vi "FipsAdjacent.vi"() -> (11 "Fips":i32[](array[numeric]))   [LabVIEW 2017] (continued)
40035\t\"Labette County, KS\"\t20099\n\"Craig County, OK\"\t40035\t\"Craig County, OK\"\t40035\n\"Craig County, OK\"\t40035\t\"Delaware County, OK\"\t40041\n\"Craig County, OK\"\t40035\t\"Mayes County, OK\"\t40097\n\"Craig County, OK\"\t40035\t\"Nowata County, OK\"\t40105\n\"Craig County, OK\"\t40035\t\"Ottawa County, OK\"\t40115\n\"Craig County, OK\"\t40035\t\"Rogers County, OK\"\t40131\n\"Creek County, OK\"\t40037\t\"Creek County, OK\"\t40037\n\"Creek County, OK\"\t40037\t\"Lincoln County, OK\"\t40081\n\"Creek County, OK\"\t40037\t\"Okfuskee County, OK\"\t40107\n\"Creek County, OK\"\t40037\t\"Okmulgee County, OK\"\t40111\n\"Creek County, OK\"\t40037\t\"Pawnee County, OK\"\t40117\n\"Creek County, OK\"\t40037\t\"Payne County, OK\"\t40119\n\"Creek County, OK\"\t40037\t\"Tulsa County, OK\"\t40143\n\"Custer County, OK\"\t40039\t\"Beckham County, OK\"\t40009\n\"Custer County, OK\"\t40039\t\"Blaine County, OK\"\t40011\n\"Custer County, OK\"\t40039\t\"Caddo County, OK\"\t40015\n\"Custer County, OK\"\t40039\t\"Custer County, OK\"\t40039\n\"Custer County, OK\"\t40039\t\"Dewey County, OK\"\t40043\n\"Custer County, OK\"\t40039\t\"Roger Mills County, OK\"\t40129\n\"Custer County, OK\"\t40039\t\"Washita County, OK\"\t40149\n\"Delaware County, OK\"\t40041\t\"Benton County, AR\"\t05007\n\"Delaware County, OK\"\t40041\t\"McDonald County, MO\"\t29119\n\"Delaware County, OK\"\t40041\t\"Adair County, OK\"\t40001\n\"Delaware County, OK\"\t40041\t\"Cherokee County, OK\"\t40021\n\"Delaware County, OK\"\t40041\t\"Craig County, OK\"\t40035\n\"Delaware County, OK\"\t40041\t\"Delaware County, OK\"\t40041\n\"Delaware County, OK\"\t40041\t\"Mayes County, OK\"\t40097\n\"Delaware County, OK\"\t40041\t\"Ottawa County, OK\"\t40115\n\"Dewey County, OK\"\t40043\t\"Blaine County, OK\"\t40011\n\"Dewey County, OK\"\t40043\t\"Custer County, OK\"\t40039\n\"Dewey County, OK\"\t40043\t\"Dewey County, OK\"\t40043\n\"Dewey County, OK\"\t40043\t\"Ellis County, OK\"\t40045\n\"Dewey County, OK\"\t40043\t\"Major County, OK\"\t40093\n\"Dewey County, OK\"\t40043\t\"Roger Mills County, OK\"\t40129\n\"Dewey County, OK\"\t40043\t\"Woodward County, OK\"\t40153\n\"Ellis County, OK\"\t40045\t\"Beaver County, OK\"\t40007\n\"Ellis County, OK\"\t40045\t\"Dewey County, OK\"\t40043\n\"Ellis County, OK\"\t40045\t\"Ellis County, OK\"\t40045\n\"Ellis County, OK\"\t40045\t\"Harper County, OK\"\t40059\n\"Ellis County, OK\"\t40045\t\"Roger Mills County, OK\"\t40129\n\"Ellis County, OK\"\t40045\t\"Woodward County, OK\"\t40153\n\"Ellis County, OK\"\t40045\t\"Hemphill County, TX\"\t48211\n\"Ellis County, OK\"\t40045\t\"Lipscomb County, TX\"\t48295\n\"Garfield County, OK\"\t40047\t\"Alfalfa County, OK\"\t40003\n\"Garfield County, OK\"\t40047\t\"Garfield County, OK\"\t40047\n\"Garfield County, OK\"\t40047\t\"Grant County, OK\"\t40053\n\"Garfield County, OK\"\t40047\t\"Kay County, OK\"\t40071\n\"Garfield County, OK\"\t40047\t\"Kingfisher County, OK\"\t40073\n\"Garfield County, OK\"\t40047\t\"Logan County, OK\"\t40083\n\"Garfield County, OK\"\t40047\t\"Major County, OK\"\t40093\n\"Garfield County, OK\"\t40047\t\"Noble County, OK\"\t40103\n\"Garvin County, OK\"\t40049\t\"Carter County, OK\"\t40019\n\"Garvin County, OK\"\t40049\t\"Garvin County, OK\"\t40049\n\"Garvin County, OK\"\t40049\t\"Grady County, OK\"\t40051\n\"Garvin County, OK\"\t40049\t\"McClain County, OK\"\t40087\n\"Garvin County, OK\"\t40049\t\"Murray County, OK\"\t40099\n\"Garvin County, OK\"\t40049\t\"Pontotoc County, OK\"\t40123\n\"Garvin County, OK\"\t40049\t\"Stephens County, OK\"\t40137\n\"Grady County, OK\"\t40051\t\"Caddo County, OK\"\t40015\n\"Grady County, OK\"\t40051\t\"Canadian County, OK\"\t40017\n\"Grady County, OK\"\t40051\t\"Comanche County, OK\"\t40031\n\"Grady County, OK\"\t40051\t\"Garvin County, OK\"\t40049\n\"Grady County, OK\"\t40051\t\"Grady County, OK\"\t40051\n\"Grady County, OK\"\t40051\t\"McClain County, OK\"\t40087\n\"Grady County, OK\"\t40051\t\"Stephens County, OK\"\t40137\n\"Grant County, OK\"\t40053\t\"Harper County, KS\"\t20077\n\"Grant County, OK\"\t40053\t\"Sumner County, KS\"\t20191\n\"Grant County, OK\"\t40053\t\"Alfalfa County, OK\"\t40003\n\"Grant County, OK\"\t40053\t\"Garfield County, OK\"\t40047\n\"Grant County, OK\"\t40053\t\"Grant County, OK\"\t40053\n\"Grant County, OK\"\t40053\t\"Kay County, OK\"\t40071\n\"Greer County, OK\"\t40055\t\"Beckham County, OK\"\t40009\n\"Greer County, OK\"\t40055\t\"Greer County, OK\"\t40055\n\"Greer County, OK\"\t40055\t\"Harmon County, OK\"\t40057\n\"Greer County, OK\"\t40055\t\"Jackson County, OK\"\t40065\n\"Greer County, OK\"\t40055\t\"Kiowa County, OK\"\t40075\n\"Harmon County, OK\"\t40057\t\"Beckham County, OK\"\t40009\n\"Harmon County, OK\"\t40057\t\"Greer County, OK\"\t40055\n\"Harmon County, OK\"\t40057\t\"Harmon County, OK\"\t40057\n\"Harmon County, OK\"\t40057\t\"Jackson County, OK\"\t40065\n\"Harmon County, OK\"\t40057\t\"Childress County, TX\"\t48075\n\"Harmon County, OK\"\t40057\t\"Collingsworth County, TX\"\t48087\n\"Harmon County, OK\"\t40057\t\"Hardeman County, TX\"\t48197\n\"Harper County, OK\"\t40059\t\"Clark County, KS\"\t20025\n\"Harper County, OK\"\t40059\t\"Comanche County, KS\"\t20033\n\"Harper County, OK\"\t40059\t\"Beaver County, OK\"\t40007\n\"Harper County, OK\"\t40059\t\"Ellis County, OK\"\t40045\n\"Harper County, OK\"\t40059\t\"Harper County, OK\"\t40059\n\"Harper County, OK\"\t40059\t\"Woods County, OK\"\t40151\n\"Harper County, OK\"\t40059\t\"Woodward County, OK\"\t40153\n\"Haskell County, OK\"\t40061\t\"Haskell County, OK\"\t40061\n\"Haskell County, OK\"\t40061\t\"Latimer County, OK\"\t40077\n\"Haskell County, OK\"\t40061\t\"Le Flore County, OK\"\t40079\n\"Haskell County, OK\"\t40061\t\"McIntosh County, OK\"\t40091\n\"Haskell County, OK\"\t40061\t\"Muskogee County, OK\"\t40101\n\"Haskell County, OK\"\t40061\t\"Pittsburg County, OK\"\t40121\n\"Haskell County, OK\"\t40061\t\"Sequoyah County, OK\"\t40135\n\"Hughes County, OK\"\t40063\t\"Coal County, OK\"\t40029\n\"Hughes County, OK\"\t40063\t\"Hughes County, OK\"\t40063\n\"Hughes County, OK\"\t40063\t\"McIntosh County, OK\"\t40091\n\"Hughes County, OK\"\t40063\t\"Okfuskee County, OK\"\t40107\n\"Hughes County, OK\"\t40063\t\"Pittsburg County, OK\"\t40121\n\"Hughes County, OK\"\t40063\t\"Pontotoc County, OK\"\t40123\n\"Hughes County, OK\"\t40063\t\"Seminole County, OK\"\t40133\n\"Jackson County, OK\"\t40065\t\"Greer County, OK\"\t40055\n\"Jackson County, OK\"\t40065\t\"Harmon County, OK\"\t40057\n\"Jackson County, OK\"\t40065\t\"Jackson County, OK\"\t40065\n\"Jackson County, OK\"\t40065\t\"Kiowa County, OK\"\t40075\n\"Jackson County, OK\"\t40065\t\"Tillman County, OK\"\t40141\n\"Jackson County, OK\"\t40065\t\"Hardeman County, TX\"\t48197\n\"Jackson County, OK\"\t40065\t\"Wilbarger County, TX\"\t48487\n\"Jefferson County, OK\"\t40067\t\"Carter County, OK\"\t40019\n\"Jefferson County, OK\"\t40067\t\"Cotton County, OK\"\t40033\n\"Jefferson County, OK\"\t40067\t\"Jefferson County, OK\"\t40067\n\"Jefferson County, OK\"\t40067\t\"Love County, OK\"\t40085\n\"Jefferson County, OK\"\t40067\t\"Stephens County, OK\"\t40137\n\"Jefferson County, OK\"\t40067\t\"Clay County, TX\"\t48077\n\"Jefferson County, OK\"\t40067\t\"Montague County, TX\"\t48337\n\"Johnston County, OK\"\t40069\t\"Atoka County, OK\"\t40005\n\"Johnston County, OK\"\t40069\t\"Bryan County, OK\"\t40013\n\"Johnston County, OK\"\t40069\t\"Carter County, OK\"\t40019\n\"Johnston County, OK\"\t40069\t\"Coal County, OK\"\t40029\n\"Johnston County, OK\"\t40069\t\"Johnston County, OK\"\t40069\n\"Johnston County, OK\"\t40069\t\"Marshall County, OK\"\t40095\n\"Johnston County, OK\"\t40069\t\"Murray County, OK\"\t40099\n\"Johnston County, OK\"\t40069\t\"Pontotoc County, OK\"\t40123\n\"Kay County, OK\"\t40071\t\"Cowley County, KS\"\t20035\n\"Kay County, OK\"\t40071\t\"Sumner County, KS\"\t20191\n\"Kay County, OK\"\t40071\t\"Garfield County, OK\"\t40047\n\"Kay County, OK\"\t40071\t\"Grant County, OK\"\t40053\n\"Kay County, OK\"\t40071\t\"Kay County, OK\"\t40071\n\"Kay County, OK\"\t40071\t\"Noble County, OK\"\t40103\n\"Kay County, OK\"\t40071\t\"Osage County, OK\"\t40113\n\"Kingfisher County, OK\"\t40073\t\"Blaine County, OK\"\t40011\n\"Kingfisher County, OK\"\t40073\t\"Canadian County, OK\"\t40017\n\"Kingfisher County, OK\"\t40073\t\"Garfield County, OK\"\t40047\n\"Kingfisher County, OK\"\t40073\t\"Kingfisher County, OK\"\t40073\n\"Kingfisher County, OK\"\t40073\t\"Logan County, OK\"\t40083\n\"Kingfisher County, OK\"\t40073\t\"Major County, OK\"\t40093\n\"Kingfisher County, OK\"\t40073\t\"Oklahoma County, OK\"\t40109\n\"Kiowa County, OK\"\t40075\t\"Beckham County, OK\"\t40009\n\"Kiowa County, OK\"\t40075\t\"Caddo County, OK\"\t40015\n\"Kiowa County, OK\"\t40075\t\"Comanche County, OK\"\t40031\n\"Kiowa County, OK\"\t40075\t\"Greer County, OK\"\t40055\n\"Kiowa County, OK\"\t40075\t\"Jackson County, OK\"\t40065\n\"Kiowa County, OK\"\t40075\t\"Kiowa County, OK\"\t40075\n\"Kiowa County, OK\"\t40075\t\"Tillman County, OK\"\t40141\n\"Kiowa County, OK\"\t40075\t\"Washita County, OK\"\t40149\n\"Latimer County, OK\"\t40077\t\"Haskell County, OK\"\t40061\n\"Latimer County, OK\"\t40077\t\"Latimer County, OK\"\t40077\n\"Latimer County, OK\"\t40077\t\"Le Flore County, OK\"\t40079\n\"Latimer County, OK\"\t40077\t\"Pittsburg County, OK\"\t40121\n\"Latimer County, OK\"\t40077\t\"Pushmataha County, OK\"\t40127\n\"Le Flore County, OK\"\t40079\t\"Polk County, AR\"\t05113\n\"Le Flore County, OK\"\t40079\t\"Scott County, AR\"\t05127\n\"Le Flore County, OK\"\t40079\t\"Sebastian County, AR\"\t05131\n\"Le Flore County, OK\"\t40079\t\"Haskell County, OK\"\t40061\n\"Le Flore County, OK\"\t40079\t\"Latimer County, OK\"\t40077\n\"Le Flore County, OK\"\t40079\t\"Le Flore County, OK\"\t40079\n\"Le Flore County, OK\"\t40079\t\"McCurtain County, OK\"\t40089\n\"Le Flore County, OK\"\t40079\t\"Pushmataha County, OK\"\t40127\n\"Le Flore County, OK\"\t40079\t\"Sequoyah County, OK\"\t40135\n\"Lincoln County, OK\"\t40081\t\"Creek County, OK\"\t40037\n\"Lincoln County, OK\"\t40081\t\"Lincoln County, OK\"\t40081\n\"Lincoln County, OK\"\t40081\t\"Logan County, OK\"\t40083\n\"Lincoln County, OK\"\t40081\t\"Okfuskee County, OK\"\t40107\n\"Lincoln County, OK\"\t40081\t\"Oklahoma County, OK\"\t40109\n\"Lincoln County, OK\"\t40081\t\"Payne County, OK\"\t40119\n\"Lincoln County, OK\"\t40081\t\"Pottawatomie County, OK\"\t40125\n\"Logan County, OK\"\t40083\t\"Canadian County, OK\"\t40017\n\"Logan County, OK\"\t40083\t\"Garfield County, OK\"\t40047\n\"Logan County, OK\"\t40083\t\"Kingfisher County, OK\"\t40073\n\"Logan County, OK\"\t40083\t\"Lincoln County, OK\"\t40081\n\"Logan County, OK\"\t40083\t\"Logan County, OK\"\t40083\n\"Logan County, OK\"\t40083\t\"Noble County, OK\"\t40103\n\"Logan County, OK\"\t40083\t\"Oklahoma County, OK\"\t40109\n\"Logan County, OK\"\t40083\t\"Payne County, OK\"\t40119\n\"Love County, OK\"\t40085\t\"Carter County, OK\"\t40019\n\"Love County, OK\"\t40085\t\"Jefferson County, OK\"\t40067\n\"Love County, OK\"\t40085\t\"Love County, OK\"\t40085\n\"Love County, OK\"\t40085\t\"Marshall County, OK\"\t40095\n\"Love County, OK\"\t40085\t\"Cooke County, TX\"\t48097\n\"Love County, OK\"\t40085\t\"Grayson County, TX\"\t48181\n\"Love County, OK\"\t40085\t\"Montague County, TX\"\t48337\n\"McClain County, OK\"\t40087\t\"Canadian County, OK\"\t40017\n\"McClain County, OK\"\t40087\t\"Cleveland County, OK\"\t40027\n\"McClain County, OK\"\t40087\t\"Garvin County, OK\"\t40049\n\"McClain County, OK\"\t40087\t\"Grady County, OK\"\t40051\n\"McClain County, OK\"\t40087\t\"McClain County, OK\"\t40087\n\"McClain County, OK\"\t40087\t\"Pontotoc County, OK\"\t40123\n\"McClain County, OK\"\t40087\t\"Pottawatomie County, OK\"\t40125\n\"McCurtain County, OK\"\t40089\t\"Little River County, AR\"\t05081\n\"McCurtain County, OK\"\t40089\t\"Polk County, AR\"\t05113\n\"McCurtain County, OK\"\t40089\t\"Sevier County, AR\"\t05133\n\"McCurtain County, OK\"\t40089\t\"Choctaw County, OK\"\t40023\n\"McCurtain County, OK\"\t40089\t\"Le Flore County, OK\"\t40079\n\"McCurtain County, OK\"\t40089\t\"McCurtain County, OK\"\t40089\n\"McCurtain County, OK\"\t40089\t\"Pushmataha County, OK\"\t40127\n\"McCurtain County, OK\"\t40089\t\"Bowie County, TX\"\t48037\n\"McCurtain County, OK\"\t40089\t\"Red River County, TX\"\t48387\n\"McIntosh County, OK\"\t40091\t\"Haskell County, OK\"\t40061\n\"McIntosh County, OK\"\t40091\t\"Hughes County, OK\"\t40063\n\"McIntosh County, OK\"\t40091\t\"McIntosh County, OK\"\t40091\n\"McIntosh County, OK\"\t40091\t\"Muskogee County, OK\"\t40101\n\"McIntosh County, OK\"\t40091\t\"Okfuskee County, OK\"\t40107\n\"McIntosh County, OK\"\t40091\t\"Okmulgee County, OK\"\t40111\n\"McIntosh County, OK\"\t40091\t\"Pittsburg County, OK\"\t40121\n\"Major County, OK\"\t40093\t\"Alfalfa County, OK\"\t40003\n\"Major County, OK\"\t40093\t\"Blaine County, OK\"\t40011\n\"Major County, OK\"\t40093\t\"Dewey County, OK\"\t40043\n\"Major County, OK\"\t40093\t\"Garfield County, OK\"\t40047\n\"Major County, OK\"\t40093\t\"Kingfisher County, OK\"\t40073\n\"Major County, OK\"\t40093\t\"Major County, OK\"\t40093\n\"Major County, OK\"\t40093\t\"Woods County, OK\"\t40151\n\"Major County, OK\"\t40093\t\"Woodward County, OK\"\t40153\n\"Marshall County, OK\"\t40095\t\"Bryan County, OK\"\t40013\n\"Marshall County, OK\"\t40095\t\"Carter County, OK\"\t40019\n\"Marshall County, OK\"\t40095\t\"Johnston County, OK\"\t40069\n\"Marshall County, OK\"\t40095\t\"Love County, OK\"\t40085\n\"Marshall County, OK\"\t40095\t\"Marshall County, OK\"\t40095\n\"Marshall County, OK\"\t40095\t\"Grayson County, TX\"\t48181\n\"Mayes County, OK\"\t40097\t\"Cherokee County, OK\"\t40021\n\"Mayes County, OK\"\t40097\t\"Craig County, OK\"\t40035\n\"Mayes County, OK\"\t40097\t\"Delaware County, OK\"\t40041\n\"Mayes County, OK\"\t40097\t\"Mayes County, OK\"\t40097\n\"Mayes County, OK\"\t40097\t\"Rogers County, OK\"\t40131\n\"Mayes County, OK\"\t40097\t\"Wagoner County, OK\"\t40145\n\"Murray County, OK\"\t40099\t\"Carter County, OK\"\t40019\n\"Murray County, OK\"\t40099\t\"Garvin County, OK\"\t40049\n\"Murray County, OK\"\t40099\t\"Johnston County, OK\"\t40069\n\"Murray County, OK\"\t40099\t\"Murray County, OK\"\t40099\n\"Murray County, OK\"\t40099\t\"Pontotoc County, OK\"\t40123\n\"Muskogee County, OK\"\t40101\t\"Cherokee County, OK\"\t40021\n\"Muskogee County, OK\"\t40101\t\"Haskell County, OK\"\t40061\n\"Muskogee County, OK\"\t40101\t\"McIntosh County, OK\"\t40091\n\"Muskogee County, OK\"\t40101\t\"Muskogee County, OK\"\t40101\n\"Muskogee County, OK\"\t40101\t\"Okmulgee County, OK\"\t40111\n\"Muskogee County, OK\"\t40101\t\"Sequoyah County, OK\"\t40135\n\"Muskogee County, OK\"\t40101\t\"Wagoner County, OK\"\t40145\n\"Noble County, OK\"\t40103\t\"Garfield County, OK\"\t40047\n\"Noble County, OK\"\t40103\t\"Kay County, OK\"\t40071\n\"Noble County, OK\"\t40103\t\"Logan County, OK\"\t40083\n\"Noble County, OK\"\t40103\t\"Noble County, OK\"\t40103\n\"Noble County, OK\"\t40103\t\"Osage County, OK\"\t40113\n\"Noble County, OK\"\t40103\t\"Pawnee County, OK\"\t40117\n\"Noble County, OK\"\t40103\t\"Payne County, OK\"\t40119\n\"Nowata County, OK\"\t40105\t\"Labette County, KS\"\t20099\n\"Nowata County, OK\"\t40105\t\"Montgomery County, KS\"\t20125\n\"Nowata County, OK\"\t40105\t\"Craig County, OK\"\t40035\n\"Nowata County, OK\"\t40105\t\"Nowata County, OK\"\t40105\n\"Nowata County, OK\"\t40105\t\"Rogers County, OK\"\t40131\n\"Nowata County, OK\"\t40105\t\"Washington County, OK\"\t40147\n\"Okfuskee County, OK\"\t40107\t\"Creek County, OK\"\t40037\n\"Okfuskee County, OK\"\t40107\t\"Hughes County, OK\"\t40063\n\"Okfuskee County, OK\"\t40107\t\"Lincoln County, OK\"\t40081\n\"Okfuskee County, OK\"\t40107\t\"McIntosh County, OK\"\t40091\n\"Okfuskee County, OK\"\t40107\t\"Okfuskee County, OK\"\t40107\n\"Okfuskee County, OK\"\t40107\t\"Okmulgee County, OK\"\t40111\n\"Okfuskee County, OK\"\t40107\t\"Pottawatomie County, OK\"\t40125\n\"Okfuskee County, OK\"\t40107\t\"Seminole County, OK\"\t40133\n\"Oklahoma County, OK\"\t40109\t\"Canadian County, OK\"\t40017\n\"Oklahoma County, OK\"\t40109\t\"Cleveland County, OK\"\t40027\n\"Oklahoma County, OK\"\t40109\t\"Kingfisher County, OK\"\t40073\n\"Oklahoma County, OK\"\t40109\t\"Lincoln County, OK\"\t40081\n\"Oklahoma County, OK\"\t40109\t\"Logan County, OK\"\t40083\n\"Oklahoma County, OK\"\t40109\t\"Oklahoma County, OK\"\t40109\n\"Oklahoma County, OK\"\t40109\t\"Pottawatomie County, OK\"\t40125\n\"Okmulgee County, OK\"\t40111\t\"Creek County, OK\"\t40037\n\"Okmulgee County, OK\"\t40111\t\"McIntosh County, OK\"\t40091\n\"Okmulgee County, OK\"\t40111\t\"Muskogee County, OK\"\t40101\n\"Okmulgee County, OK\"\t40111\t\"Okfuskee County, OK\"\t40107\n\"Okmulgee County, OK\"\t40111\t\"Okmulgee County, OK\"\t40111\n\"Okmulgee County, OK\"\t40111\t\"Tulsa County, OK\"\t40143\n\"Okmulgee County, OK\"\t40111\t\"Wagoner County, OK\"\t40145\n\"Osage County, OK\"\t40113\t\"Chautauqua County, KS\"\t20019\n\"Osage County, OK\"\t40113\t\"Cowley County, KS\"\t20035\n\"Osage County, OK\"\t40113\t\"Kay County, OK\"\t40071\n\"Osage County, OK\"\t40113\t\"Noble County, OK\"\t40103\n\"Osage County, OK\"\t40113\t\"Osage County, OK\"\t40113\n\"Osage County, OK\"\t40113\t\"Pawnee County, OK\"\t40117\n\"Osage County, OK\"\t40113\t\"Tulsa County, OK\"\t40143\n\"Osage County, OK\"\t40113\t\"Washington County, OK\"\t40147\n\"Ottawa County, OK\"\t40115\t\"Cherokee County, KS\"\t20021\n\"Ottawa County, OK\"\t40115\t\"McDonald County, MO\"\t29119\n\"Ottawa County, OK\"\t40115\t\"Newton County, MO\"\t29145\n\"Ottawa County, OK\"\t40115\t\"Craig County, OK\"\t40035\n\"Ottawa County, OK\"\t40115\t\"Delaware County, OK\"\t40041\n\"Ottawa County, OK\"\t40115\t\"Ottawa County, OK\"\t40115\n\"Pawnee County, OK\"\t40117\t\"Creek County, OK\"\t40037\n\"Pawnee County, OK\"\t40117\t\"Noble County, OK\"\t40103\n\"Pawnee County, OK\"\t40117\t\"Osage County, OK\"\t40113\n\"Pawnee County, OK\"\t40117\t\"Pawnee County, OK\"\t40117\n\"Pawnee County, OK\"\t40117\t\"Payne County, OK\"\t40119\n\"Pawnee County, OK\"\t40117\t\"Tulsa County, OK\"\t40143\n\"Payne County, OK\"\t40119\t\"Creek County, OK\"\t40037\n\"Payne County, OK\"\t40119\t\"Lincoln County, OK\"\t40081\n\"Payne County, OK\"\t40119\t\"Logan County, OK\"\t40083\n\"Payne County, OK\"\t40119\t\"Noble County, OK\"\t40103\n\"Payne County, OK\"\t40119\t\"Pawnee County, OK\"\t40117\n\"Payne County, OK\"\t40119\t\"Payne County, OK\"\t40119\n\"Pittsburg County, OK\"\t40121\t\"Atoka County, OK\"\t40005\n\"Pittsburg County, OK\"\t40121\t\"Coal County, OK\"\t40029\n\"Pittsburg County, OK\"\t40121\t\"Haskell County, OK\"\t40061\n\"Pittsburg County, OK\"\t40121\t\"Hughes County, OK\"\t40063\n\"Pittsburg County, OK\"\t40121\t\"Latimer County, OK\"\t40077\n\"Pittsburg County, OK\"\t40121\t\"McIntosh County, OK\"\t40091\n\"Pittsburg County, OK\"\t40121\t\"Pittsburg County, OK\"\t40121\n\"Pittsburg County, OK\"\t40121\t\"Pushmataha County, OK\"\t40127\n\"Pontotoc County, OK\"\t40123\t\"Coal County, OK\"\t40029\n\"Pontotoc County, OK\"\t40123\t\"Garvin County, OK\"\t40049\n\"Pontotoc County, OK\"\t40123\t\"Hughes County, OK\"\t40063\n\"Pontotoc County, OK\"\t40123\t\"Johnston County, OK\"\t40069\n\"Pontotoc County, OK\"\t40123\t\"McClain County, OK\"\t40087\n\"Pontotoc County, OK\"\t40123\t\"Murray County, OK\"\t40099\n\"Pontotoc County, OK\"\t40123\t\"Pontotoc County, OK\"\t40123\n\"Pontotoc County, OK\"\t40123\t\"Pottawatomie County, OK\"\t40125\n\"Pontotoc County, OK\"\t40123\t\"Seminole County, OK\"\t40133\n\"Pottawatomie County, OK\"\t40125\t\"Cleveland County, OK\"\t40027\n\"Pottawatomie County, OK\"\t40125\t\"Lincoln County, OK\"\t40081\n\"Pottawatomie County, OK\"\t40125\t\"McClain County, OK\"\t40087\n\"Pottawatomie County, OK\"\t40125\t\"Okfuskee County, OK\"\t40107\n\"Pottawatomie County, OK\"\t40125\t\"Oklahoma County, OK\"\t40109\n\"Pottawatomie County, OK\"\t40125\t\"Pontotoc County, OK\"\t40123\n\"Pottawatomie County, OK\"\t40125\t\"Pottawatomie County, OK\"\t40125\n\"Pottawatomie County, OK\"\t40125\t\"Seminole County, OK\"\t40133\n\"Pushmataha County, OK\"\t40127\t\"Atoka County, OK\"\t40005\n\"Pushmataha County, OK\"\t40127\t\"Choctaw County, OK\"\t40023\n\"Pushmataha County, OK\"\t40127\t\"Latimer County, OK\"\t40077\n\"Pushmataha County, OK\"\t40127\t\"Le Flore County, OK\"\t40079\n\"Pushmataha County, OK\"\t40127\t\"McCurtain County, OK\"\t40089\n\"Pushmataha County, OK\"\t40127\t\"Pittsburg County, OK\"\t40121\n\"Pushmataha County, OK\"\t40127\t\"Pushmataha County, OK\"\t40127\n\"Roger Mills County, OK\"\t40129\t\"Beckham County, OK\"\t40009\n\"Roger Mills County, OK\"\t40129\t\"Custer County, OK\"\t40039\n\"Roger Mills County, OK\"\t40129\t\"Dewey County, OK\"\t40043\n\"Roger Mills County, OK\"\t40129\t\"Ellis County, OK\"\t40045\n\"Roger Mills County, OK\"\t40129\t\"Roger Mills County, OK\"\t40129\n\"Roger Mills County, OK\"\t40129\t\"Hemphill County, TX\"\t48211\n\"Roger Mills County, OK\"\t40129\t\"Wheeler County, TX\"\t48483\n\"Rogers County, OK\"\t40131\t\"Craig County, OK\"\t40035\n\"Rogers County, OK\"\t40131\t\"Mayes County, OK\"\t40097\n\"Rogers County, OK\"\t40131\t\"Nowata County, OK\"\t40105\n\"Rogers County, OK\"\t40131\t\"Rogers County, OK\"\t40131\n\"Rogers County, OK\"\t40131\t\"Tulsa County, OK\"\t40143\n\"Rogers County, OK\"\t40131\t\"Wagoner County, OK\"\t40145\n\"Rogers County, OK\"\t40131\t\"Washington County, OK\"\t40147\n\"Seminole County, OK\"\t40133\t\"Hughes County, OK\"\t40063\n\"Seminole County, OK\"\t40133\t\"Okfuskee County, OK\"\t40107\n\"Seminole County, OK\"\t40133\t\"Pontotoc County, OK\"\t40123\n\"Seminole County, OK\"\t40133\t\"Pottawatomie County, OK\"\t40125\n\"Seminole County, OK\"\t40133\t\"Seminole County, OK\"\t40133\n\"Sequoyah County, OK\"\t40135\t\"Crawford County, AR\"\t05033\n\"Sequoyah County, OK\"\t40135\t\"Sebastian County, AR\"\t05131\n\"Sequoyah County, OK\"\t40135\t\"Adair County, OK\"\t40001\n\"Sequoyah County, OK\"\t40135\t\"Cherokee County, OK\"\t40021\n\"Sequoyah County, OK\"\t40135\t\"Haskell County, OK\"\t40061\n\"Sequoyah County, OK\"\t40135\t\"Le Flore County, OK\"\t40079\n\"Sequoyah County, OK\"\t40135\t\"Muskogee County, OK\"\t40101\n\"Sequoyah County, OK\"\t40135\t\"Sequoyah County, OK\"\t40135\n\"Stephens County, OK\"\t40137\t\"Carter County, OK\"\t40019\n\"Stephens County, OK\"\t40137\t\"Comanche County, OK\"\t40031\n\"Stephens County, OK\"\t40137\t\"Cotton County, OK\"\t40033\n\"Stephens County, OK\"\t40137\t\"Garvin County, OK\"\t40049\n\"Stephens County, OK\"\t40137\t\"Grady County, OK\"\t40051\n\"Stephens County, OK\"\t40137\t\"Jefferson County, OK\"\t40067\n\"Stephens County, OK\"\t40137\t\"Stephens County, OK\"\t40137\n\"Texas County, OK\"\t40139\t\"Morton County, KS\"\t20129\n\"Texas County, OK\"\t40139\t\"Seward County, KS\"\t20175\n\"Texas County, OK\"\t40139\t\"Stevens County, KS\"\t20189\n\"Texas County, OK\"\t40139\t\"Beaver County, OK\"\t40007\n\"Texas County, OK\"\t40139\t\"Cimarron County, OK\"\t40025\n\"Texas County, OK\"\t40139\t\"Texas County, OK\"\t40139\n\"Texas County, OK\"\t40139\t\"Hansford County, TX\"\t48195\n\"Texas County, OK\"\t40139\t\"Ochiltree County, TX\"\t48357\n\"Texas County, OK\"\t40139\t\"Sherman County, TX\"\t48421\n\"Tillman County, OK\"\t40141\t\"Comanche County, OK\"\t40031\n\"Tillman County, OK\"\t40141\t\"Cotton County, OK\"\t40033\n\"Tillman County, OK\"\t40141\t\"Jackson County, OK\"\t40065\n\"Tillman County, OK\"\t40141\t\"Kiowa County, OK\"\t40075\n\"Tillman County, OK\"\t40141\t\"Tillman County, OK\"\t40141\n\"Tillman County, OK\"\t40141\t\"Wichita County, TX\"\t48485\n\"Tillman County, OK\"\t40141\t\"Wilbarger County, TX\"\t48487\n\"Tulsa County, OK\"\t40143\t\"Creek County, OK\"\t40037\n\"Tulsa County, OK\"\t40143\t\"Okmulgee County, OK\"\t40111\n\"Tulsa County, OK\"\t40143\t\"Osage County, OK\"\t40113\n\"Tulsa County, OK\"\t40143\t\"Pawnee County, OK\"\t40117\n\"Tulsa County, OK\"\t40143\t\"Rogers County, OK\"\t40131\n\"Tulsa County, OK\"\t40143\t\"Tulsa County, OK\"\t40143\n\"Tulsa County, OK\"\t40143\t\"Wagoner County, OK\"\t40145\n\"Tulsa County, OK\"\t40143\t\"Washington County, OK\"\t40147\n\"Wagoner County, OK\"\t40145\t\"Cherokee County, OK\"\t40021\n\"Wagoner County, OK\"\t40145\t\"Mayes County, OK\"\t40097\n\"Wagoner County, OK\"\t40145\t\"Muskogee County, OK\"\t40101\n\"Wagoner County, OK\"\t40145\t\"Okmulgee County, OK\"\t40111\n\"Wagoner County, OK\"\t40145\t\"Rogers County, OK\"\t40131\n\"Wagoner County, OK\"\t40145\t\"Tulsa County, OK\"\t40143\n\"Wagoner County, OK\"\t40145\t\"Wagoner County, OK\"\t40145\n\"Washington County, OK\"\t40147\t\"Chautauqua County, KS\"\t20019\n\"Washington County, OK\"\t40147\t\"Montgomery County, KS\"\t20125\n\"Washington County, OK\"\t40147\t\"Nowata County, OK\"\t40105\n\"Washington County, OK\"\t40147\t\"Osage County, OK\"\t40113\n\"Washington County, OK\"\t40147\t\"Rogers County, OK\"\t40131\n\"Washington County, OK\"\t40147\t\"Tulsa County, OK\"\t40143\n\"Washington County, OK\"\t40147\t\"Washington County, OK\"\t40147\n\"Washita County, OK\"\t40149\t\"Beckham County, OK\"\t40009\n\"Washita County, OK\"\t40149\t\"Caddo County, OK\"\t40015\n\"Washita County, OK\"\t40149\t\"Custer County, OK\"\t40039\n\"Washita County, OK\"\t40149\t\"Kiowa County, OK\"\t40075\n\"Washita County, OK\"\t40149\t\"Washita County, OK\"\t40149\n\"Woods County, OK\"\t40151\t\"Barber County, KS\"\t20007\n\"Woods County, OK\"\t40151\t\"Comanche County, KS\"\t20033\n\"Woods County, OK\"\t40151\t\"Alfalfa County, OK\"\t40003\n\"Woods County, OK\"\t40151\t\"Harper County, OK\"\t40059\n\"Woods County, OK\"\t40151\t\"Major County, OK\"\t40093\n\"Woods County, OK\"\t40151\t\"Woods County, OK\"\t40151\n\"Woods County, OK\"\t40151\t\"Woodward County, OK\"\t40153\n\"Woodward County, OK\"\t40153\t\"Dewey County, OK\"\t40043\n\"Woodward County, OK\"\t40153\t\"Ellis County, OK\"\t40045\n\"Woodward County, OK\"\t40153\t\"Harper County, OK\"\t40059\n\"Woodward County, OK\"\t40153\t\"Major County, OK\"\t40093\n\"Woodward County, OK\"\t40153\t\"Woods County, OK\"\t40151\n\"Woodward County, OK\"\t40153\t\"Woodward County, OK\"\t40153\n\"Baker County, OR\"\t41001\t\"Adams County, ID\"\t16003\n\"Baker County, OR\"\t41001\t\"Washington County, ID\"\t16087\n\"Baker County, OR\"\t41001\t\"Baker County, OR\"\t41001\n\"Baker County, OR\"\t41001\t\"Grant County, OR\"\t41023\n\"Baker County, OR\"\t41001\t\"Malheur County, OR\"\t41045\n\"Baker County, OR\"\t41001\t\"Union County, OR\"\t41061\n\"Baker County, OR\"\t41001\t\"Wallowa County, OR\"\t41063\n\"Benton County, OR\"\t41003\t\"Benton County, OR\"\t41003\n\"Benton County, OR\"\t41003\t\"Lane County, OR\"\t41039\n\"Benton County, OR\"\t41003\t\"Lincoln County, OR\"\t41041\n\"Benton County, OR\"\t41003\t\"Linn County, OR\"\t41043\n\"Benton County, OR\"\t41003\t\"Polk County, OR\"\t41053\n\"Clackamas County, OR\"\t41005\t\"Clackamas County, OR\"\t41005\n\"Clackamas County, OR\"\t41005\t\"Hood River County, OR\"\t41027\n\"Clackamas County, OR\"\t41005\t\"Marion County, OR\"\t41047\n\"Clackamas County, OR\"\t41005\t\"Multnomah County, OR\"\t41051\n\"Clackamas County, OR\"\t41005\t\"Wasco County, OR\"\t41065\n\"Clackamas County, OR\"\t41005\t\"Washington County, OR\"\t41067\n\"Clackamas County, OR\"\t41005\t\"Yamhill County, OR\"\t41071\n\"Clatsop County, OR\"\t41007\t\"Clatsop County, OR\"\t41007\n\"Clatsop County, OR\"\t41007\t\"Columbia County, OR\"\t41009\n\"Clatsop County, OR\"\t41007\t\"Tillamook County, OR\"\t41057\n\"Clatsop County, OR\"\t41007\t\"Washington County, OR\"\t41067\n\"Clatsop County, OR\"\t41007\t\"Pacific County, WA\"\t53049\n\"Clatsop County, OR\"\t41007\t\"Wahkiakum County, WA\"\t53069\n\"Columbia County, OR\"\t41009\t\"Clatsop County, OR\"\t41007\n\"Columbia County, OR\"\t41009\t\"Columbia County, OR\"\t41009\n\"Columbia County, OR\"\t41009\t\"Multnomah County, OR\"\t41051\n\"Columbia County, OR\"\t41009\t\"Tillamook County, OR\"\t41057\n\"Columbia County, OR\"\t41009\t\"Washington County, OR\"\t41067\n\"Columbia County, OR\"\t41009\t\"Clark County, WA\"\t53011\n\"Columbia County, OR\"\t41009\t\"Cowlitz County, WA\"\t53015\n\"Columbia County, OR\"\t41009\t\"Wahkiakum County, WA\"\t53069\n\"Coos County, OR\"\t41011\t\"Coos County, OR\"\t41011\n\"Coos County, OR\"\t41011\t\"Curry County, OR\"\t41015\n\"Coos County, OR\"\t41011\t\"Douglas County, OR\"\t41019\n\"Crook County, OR\"\t41013\t\"Crook County, OR\"\t41013\n\"Crook County, OR\"\t41013\t\"Deschutes County, OR\"\t41017\n\"Crook County, OR\"\t41013\t\"Grant County, OR\"\t41023\n\"Crook County, OR\"\t41013\t\"Harney County, OR\"\t41025\n\"Crook County, OR\"\t41013\t\"Jefferson County, OR\"\t41031\n\"Crook County, OR\"\t41013\t\"Wheeler County, OR\"\t41069\n\"Curry County, OR\"\t41015\t\"Del Norte County, CA\"\t06015\n\"Curry County, OR\"\t41015\t\"Coos County, OR\"\t41011\n\"Curry County, OR\"\t41015\t\"Curry County, OR\"\t41015\n\"Curry County, OR\"\t41015\t\"Douglas County, OR\"\t41019\n\"Curry County, OR\"\t41015\t\"Josephine County, OR\"\t41033\n\"Deschutes County, OR\"\t41017\t\"Crook County, OR\"\t41013\n\"Deschutes County, OR\"\t41017\t\"Deschutes County, OR\"\t41017\n\"Deschutes County, OR\"\t41017\t\"Harney County, OR\"\t41025\n\"Deschutes County, OR\"\t41017\t\"Jefferson County, OR\"\t41031\n\"Deschutes County, OR\"\t41017\t\"Klamath County, OR\"\t41035\n\"Deschutes County, OR\"\t41017\t\"Lake County, OR\"\t41037\n\"Deschutes County, OR\"\t41017\t\"Lane County, OR\"\t41039\n\"Deschutes County, OR\"\t41017\t\"Linn County, OR\"\t41043\n\"Douglas County, OR\"\t41019\t\"Coos County, OR\"\t41011\n\"Douglas County, OR\"\t41019\t\"Curry County, OR\"\t41015\n\"Douglas County, OR\"\t41019\t\"Douglas County, OR\"\t41019\n\"Douglas County, OR\"\t41019\t\"Jackson County, OR\"\t41029\n\"Douglas County, OR\"\t41019\t\"Josephine County, OR\"\t41033\n\"Douglas County, OR\"\t41019\t\"Klamath County, OR\"\t41035\n\"Douglas County, OR\"\t41019\t\"Lane County, OR\"\t41039\n\"Gilliam County, OR\"\t41021\t\"Gilliam County, OR\"\t41021\n\"Gilliam County, OR\"\t41021\t\"Morrow County, OR\"\t41049\n\"Gilliam County, OR\"\t41021\t\"Sherman County, OR\"\t41055\n\"Gilliam County, OR\"\t41021\t\"Wasco County, OR\"\t41065\n\"Gilliam County, OR\"\t41021\t\"Wheeler County, OR\"\t41069\n\"Gilliam County, OR\"\t41021\t\"Klickitat County, WA\"\t53039\n\"Grant County, OR\"\t41023\t\"Baker County, OR\"\t41001\n\"Grant County, OR\"\t41023\t\"Crook County, OR\"\t41013\n\"Grant County, OR\"\t41023\t\"Grant County, OR\"\t41023\n\"Grant County, OR\"\t41023\t\"Harney County, OR\"\t41025\n\"Grant County, OR\"\t41023\t\"Malheur County, OR\"\t41045\n\"Grant County, OR\"\t41023\t\"Morrow County, OR\"\t41049\n\"Grant County, OR\"\t41023\t\"Umatilla County, OR\"\t41059\n\"Grant County, OR\"\t41023\t\"Union County, OR\"\t41061\n\"Grant County, OR\"\t41023\t\"Wheeler County, OR\"\t41069\n\"Harney County, OR\"\t41025\t\"Humboldt County, NV\"\t32013\n\"Harney County, OR\"\t41025\t\"Washoe County, NV\"\t32031\n\"Harney County, OR\"\t41025\t\"Crook County, OR\"\t41013\n\"Harney County, OR\"\t41025\t\"Deschutes County, OR\"\t41017\n\"Harney County, OR\"\t41025\t\"Grant County, OR\"\t41023\n\"Harney County, OR\"\t41025\t\"Harney County, OR\"\t41025\n\"Harney County, OR\"\t41025\t\"Lake County, OR\"\t41037\n\"Harney County, OR\"\t41025\t\"Malheur County, OR\"\t41045\n\"Hood River County, OR\"\t41027\t\"Clackamas County, OR\"\t41005\n\"Hood River County, OR\"\t41027\t\"Hood River County, OR\"\t41027\n\"Hood River County, OR\"\t41027\t\"Multnomah County, OR\"\t41051\n\"Hood River County, OR\"\t41027\t\"Wasco County, OR\"\t41065\n\"Hood River County, OR\"\t41027\t\"Klickitat County, WA\"\t53039\n\"Hood River County, OR\"\t41027\t\"Skamania County, WA\"\t53059\n\"Jackson County, OR\"\t41029\t\"Siskiyou County, CA\"\t06093\n\"Jackson County, OR\"\t41029\t\"Douglas County, OR\"\t41019\n\"Jackson County, OR\"\t41029\t\"Jackson County, OR\"\t41029\n\"Jackson County, OR\"\t41029\t\"Josephine County, OR\"\t41033\n\"Jackson County, OR\"\t41029\t\"Klamath County, OR\"\t41035\n\"Jefferson County, OR\"\t41031\t\"Crook County, OR\"\t41013\n\"Jefferson County, OR\"\t41031\t\"Deschutes County, OR\"\t41017\n\"Jefferson County, OR\"\t41031\t\"Jefferson County, OR\"\t41031\n\"Jefferson County, OR\"\t41031\t\"Linn County, OR\"\t41043\n\"Jefferson County, OR\"\t41031\t\"Marion County, OR\"\t41047\n\"Jefferson County, OR\"\t41031\t\"Wasco County, OR\"\t41065\n\"Jefferson County, OR\"\t41031\t\"Wheeler County, OR\"\t41069\n\"Josephine County, OR\"\t41033\t\"Del Norte County, CA\"\t06015\n\"Josephine County, OR\"\t41033\t\"Siskiyou County, CA\"\t06093\n\"Josephine County, OR\"\t41033\t\"Curry County, OR\"\t41015\n\"Josephine County, OR\"\t41033\t\"Douglas County, OR\"\t41019\n\"Josephine County, OR\"\t41033\t\"Jackson County, OR\"\t41029\n\"Josephine County, OR\"\t41033\t\"Josephine County, OR\"\t41033\n\"Klamath County, OR\"\t41035\t\"Modoc County, CA\"\t06049\n\"Klamath County, OR\"\t41035\t\"Siskiyou County, CA\"\t06093\n\"Klamath County, OR\"\t41035\t\"Deschutes County, OR\"\t41017\n\"Klamath County, OR\"\t41035\t\"Douglas County, OR\"\t41019\n\"Klamath County, OR\"\t41035\t\"Jackson County, OR\"\t41029\n\"Klamath County, OR\"\t41035\t\"Klamath County, OR\"\t41035\n\"Klamath County, OR\"\t41035\t\"Lake County, OR\"\t41037\n\"Klamath County, OR\"\t41035\t\"Lane County, OR\"\t41039\n\"Lake County, OR\"\t41037\t\"Modoc County, CA\"\t06049\n\"Lake County, OR\"\t41037\t\"Washoe County, NV\"\t32031\n\"Lake County, OR\"\t41037\t\"Deschutes County, OR\"\t41017\n\"Lake County, OR\"\t41037\t\"Harney County, OR\"\t41025\n\"Lake County, OR\"\t41037\t\"Klamath County, OR\"\t41035\n\"Lake County, OR\"\t41037\t\"Lake County, OR\"\t41037\n\"Lane County, OR\"\t41039\t\"Benton County, OR\"\t41003\n\"Lane County, OR\"\t41039\t\"Deschutes County, OR\"\t41017\n\"Lane County, OR\"\t41039\t\"Douglas County, OR\"\t41019\n\"Lane County, OR\"\t41039\t\"Klamath County, OR\"\t41035\n\"Lane County, OR\"\t41039\t\"Lane County, OR\"\t41039\n\"Lane County, OR\"\t41039\t\"Lincoln County, OR\"\t41041\n\"Lane County, OR\"\t41039\t\"Linn County, OR\"\t41043\n\"Lincoln County, OR\"\t41041\t\"Benton County, OR\"\t41003\n\"Lincoln County, OR\"\t41041\t\"Lane County, OR\"\t41039\n\"Lincoln County, OR\"\t41041\t\"Lincoln County, OR\"\t41041\n\"Lincoln County, OR\"\t41041\t\"Polk County, OR\"\t41053\n\"Lincoln County, OR\"\t41041\t\"Tillamook County, OR\"\t41057\n\"Linn County, OR\"\t41043\t\"Benton County, OR\"\t41003\n\"Linn County, OR\"\t41043\t\"Deschutes County, OR\"\t41017\n\"Linn County, OR\"\t41043\t\"Jefferson County, OR\"\t41031\n\"Linn County, OR\"\t41043\t\"Lane County, OR\"\t41039\n\"Linn County, OR\"\t41043\t\"Linn County, OR\"\t41043\n\"Linn County, OR\"\t41043\t\"Marion County, OR\"\t41047\n\"Linn County, OR\"\t41043\t\"Polk County, OR\"\t41053\n\"Malheur County, OR\"\t41045\t\"Canyon County, ID\"\t16027\n\"Malheur County, OR\"\t41045\t\"Owyhee County, ID\"\t16073\n\"Malheur County, OR\"\t41045\t\"Payette County, ID\"\t16075\n\"Malheur County, OR\"\t41045\t\"Washington County, ID\"\t16087\n\"Malheur County, OR\"\t41045\t\"Humboldt County, NV\"\t32013\n\"Malheur County, OR\"\t41045\t\"Baker County, OR\"\t41001\n\"Malheur County, OR\"\t41045\t\"Grant County, OR\"\t41023\n\"Malheur County, OR\"\t41045\t\"Harney County, OR\"\t41025\n\"Malheur County, OR\"\t41045\t\"Malheur County, OR\"\t41045\n\"Marion County, OR\"\t41047\t\"Clackamas County, OR\"\t41005\n\"Marion County, OR\"\t41047\t\"Jefferson County, OR\"\t41031\n\"Marion County, OR\"\t41047\t\"Linn County, OR\"\t41043\n\"Marion County, OR\"\t41047\t\"Marion County, OR\"\t41047\n\"Marion County, OR\"\t41047\t\"Polk County, OR\"\t41053\n\"Marion County, OR\"\t41047\t\"Wasco County, OR\"\t41065\n\"Marion County, OR\"\t41047\t\"Yamhill County, OR\"\t41071\n\"Morrow County, OR\"\t41049\t\"Gilliam County, OR\"\t41021\n\"Morrow County, OR\"\t41049\t\"Grant County, OR\"\t41023\n\"Morrow County, OR\"\t41049\t\"Morrow County, OR\"\t41049\n\"Morrow County, OR\"\t41049\t\"Umatilla County, OR\"\t41059\n\"Morrow County, OR\"\t41049\t\"Wheeler County, OR\"\t41069\n\"Morrow County, OR\"\t41049\t\"Benton County, WA\"\t53005\n\"Morrow County, OR\"\t41049\t\"Klickitat County, WA\"\t53039\n\"Multnomah County, OR\"\t41051\t\"Clackamas County, OR\"\t41005\n\"Multnomah County, OR\"\t41051\t\"Columbia County, OR\"\t41009\n\"Multnomah County, OR\"\t41051\t\"Hood River County, OR\"\t41027\n\"Multnomah County, OR\"\t41051\t\"Multnomah County, OR\"\t41051\n\"Multnomah County, OR\"\t41051\t\"Washington County, OR\"\t41067\n\"Multnomah County, OR\"\t41051\t\"Clark County, WA\"\t53011\n\"Multnomah County, OR\"\t41051\t\"Skamania County, WA\"\t53059\n\"Polk County, OR\"\t41053\t\"Benton County, OR\"\t41003\n\"Polk County, OR\"\t41053\t\"Lincoln County, OR\"\t41041\n\"Polk County, OR\"\t41053\t\"Linn County, OR\"\t41043\n\"Polk County, OR\"\t41053\t\"Marion County, OR\"\t41047\n\"Polk County, OR\"\t41053\t\"Polk County, OR\"\t41053\n\"Polk County, OR\"\t41053\t\"Tillamook County, OR\"\t41057\n\"Polk County, OR\"\t41053\t\"Yamhill County, OR\"\t41071\n\"Sherman County, OR\"\t41055\t\"Gilliam County, OR\"\t41021\n\"Sherman County, OR\"\t41055\t\"Sherman County, OR\"\t41055\n\"Sherman County, OR\"\t41055\t\"Wasco County, OR\"\t41065\n\"Sherman County, OR\"\t41055\t\"Klickitat County, WA\"\t53039\n\"Tillamook County, OR\"\t41057\t\"Clatsop County, OR\"\t41007\n\"Tillamook County, OR\"\t41057\t\"Columbia County, OR\"\t41009\n\"Tillamook County, OR\"\t41057\t\"Lincoln County, OR\"\t41041\n\"Tillamook County, OR\"\t41057\t\"Polk County, OR\"\t41053\n\"Tillamook County, OR\"\t41057\t\"Tillamook County, OR\"\t41057\n\"Tillamook County, OR\"\t41057\t\"Washington County, OR\"\t41067\n\"Tillamook County, OR\"\t41057\t\"Yamhill County, OR\"\t41071\n\"Umatilla County, OR\"\t41059\t\"Grant County, OR\"\t41023\n\"Umatilla County, OR\"\t41059\t\"Morrow County, OR\"\t41049\n\"Umatilla County, OR\"\t41059\t\"Umatilla County, OR\"\t41059\n\"Umatilla County, OR\"\t41059\t\"Union County, OR\"\t41061\n\"Umatilla County, OR\"\t41059\t\"Wallowa County, OR\"\t41063\n\"Umatilla County, OR\"\t41059\t\"Benton County, WA\"\t53005\n\"Umatilla County, OR\"\t41059\t\"Columbia County, WA\"\t53013\n\"Umatilla County, OR\"\t41059\t\"Walla Walla County, WA\"\t53071\n\"Union County, OR\"\t41061\t\"Baker County, OR\"\t41001\n\"Union County, OR\"\t41061\t\"Grant County, OR\"\t41023\n\"Union County, OR\"\t41061\t\"Umatilla County, OR\"\t41059\n\"Union County, OR\"\t41061\t\"Union County, OR\"\t41061\n\"Union County, OR\"\t41061\t\"Wallowa County, OR\"\t41063\n\"Wallowa County, OR\"\t41063\t\"Adams County, ID\"\t16003\n\"Wallowa County, OR\"\t41063\t\"Idaho County, ID\"\t16049\n\"Wallowa County, OR\"\t41063\t\"Nez Perce County, ID\"\t16069\n\"Wallowa County, OR\"\t41063\t\"Baker County, OR\"\t41001\n\"Wallowa County, OR\"\t41063\t\"Umatilla County, OR\"\t41059\n\"Wallowa County, OR\"\t41063\t\"Union County, OR\"\t41061\n\"Wallowa County, OR\"\t41063\t\"Wallowa County, OR\"\t41063\n\"Wallowa County, OR\"\t41063\t\"Asotin County, WA\"\t53003\n\"Wallowa County, OR\"\t41063\t\"Columbia County, WA\"\t53013\n\"Wallowa County, OR\"\t41063\t\"Garfield County, WA\"\t53023\n\"Wasco County, OR\"\t41065\t\"Clackamas County, OR\"\t41005\n\"Wasco County, OR\"\t41065\t\"Gilliam County, OR\"\t41021\n\"Wasco County, OR\"\t41065\t\"Hood River County, OR\"\t41027\n\"Wasco County, OR\"\t41065\t\"Jefferson County, OR\"\t41031\n\"Wasco County, OR\"\t41065\t\"Marion County, OR\"\t41047\n\"Wasco County, OR\"\t41065\t\"Sherman County, OR\"\t41055\n\"Wasco County, OR\"\t41065\t\"Wasco County, OR\"\t41065\n\"Wasco County, OR\"\t41065\t\"Wheeler County, OR\"\t41069\n\"Wasco County, OR\"\t41065\t\"Klickitat County, WA\"\t53039\n\"Washington County, OR\"\t41067\t\"Clackamas County, OR\"\t41005\n\"Washington County, OR\"\t41067\t\"Clatsop County, OR\"\t41007\n\"Washington County, OR\"\t41067\t\"Columbia County, OR\"\t41009\n\"Washington County, OR\"\t41067\t\"Multnomah County, OR\"\t41051\n\"Washington County, OR\"\t
